vi "Constructor.vi"(7 "FP_Control_Flag":string="UI_", 8 "error in":errorcluster, 10 "UI_Ref":refnum<vi>, 11 "UI_Manager in":refnum<class "UI_Library.lvclass">) -> (0 "error out":errorcluster, 2 "UI_Queue":refnum<queue>, 3 "UI_Manager out":refnum<class "UI_Library.lvclass">)   [LabVIEW 2018, in "UI_Library.lvlib" / "UI_Library.lvclass"]
doc: "Initialize Class queue and properties"
uses:
  UI_Library.lvclass
  UI_Library.lvclass/UI_Library.ctl
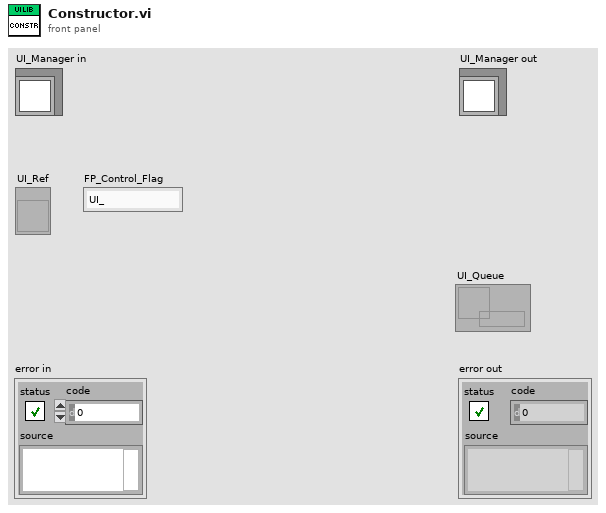
[diagram p1: front panel]
types:
  T1 = cluster{"UIEvent":string, "EventData":variant, "Register":bool}
  T2 = typedef "UI_Library.lvlib/UI_RefCluster.ctl" = cluster{"UI Ctrl Names":string[], "UI Ctrl DataType":T3[], "UI Ctrl Refs":refnum<vi>[]}
  T3 = typedef "NI_Data Type.lvlib/Data Type.ctl" = enum8{"Invalid Type", "Void", "I8", "I16", "I32", "I64", "U8", "U16", "U32", "U64", "Single Float", "Double Float", "Extended Float", "Single Complex", "Double Complex", "Extended Complex", "Enum U8", "Enum U16", "Enum U32", "Enum U64", "Single Float With Unit", "Double Float With Unit", "Extended Float With Unit", "Single Complex with Unit", "Double Complex with Unit", "Extended Complex with Unit", "Boolean", "String", "Path", "Picture", "Tag", "Array", "Cluster", "Variant", "LV Variant", "Waveform", "Timestamp", "Digital Waveform", "Digital Data", "ExpressData", "Refnum", "External Data", "VI", "Poly VI", "LabVIEW Class Instance", "Fixed Point", "Set Collection", "Map Collection"}
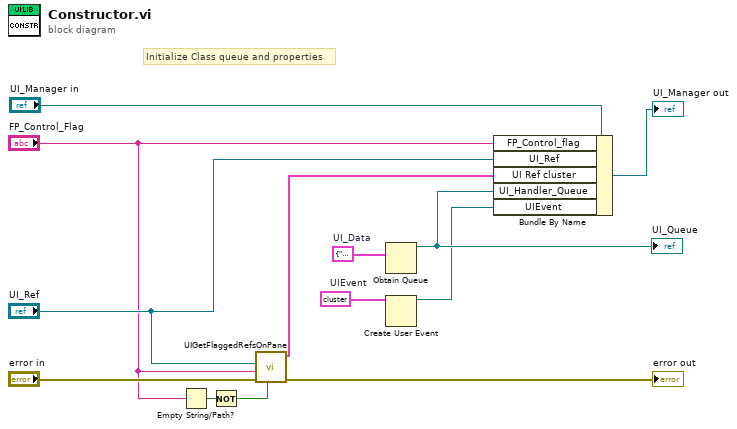
[diagram p0: block diagram]
diagram:
  w4 = T1 {"UIEvent"="", "EventData"=variant, "Register"=FALSE}  # UIEvent
  w12 = cluster{"cmd":string, "data":variant} {"cmd"="", "data"=variant}  # UI_Data
  # "Initialize Class queue and properties"
  n1 = Empty String/Path?(string/path="FP_Control_Flag") -> (empty?=w8:bool)
  n2 = Not(x=w8) -> (.not. x?=w6:bool)
  n3 = call "UIGetFlaggedRefsOnPane.vi"("Check Flag (T)"=w6, "error in"="error in", "Flag"="FP_Control_Flag", "VI Ref"="UI_Ref") -> ("error out"=→"error out":errorcluster, "UI Ref cluster out"=w5:T2)  [unwired: 6 in]
  n4 = Obtain Queue(element data type=w12) -> (queue out=w3:refnum<queue>)  [unwired: 4 in, 2 out]
  "UI_Queue" <- w3
  n5 = Create User Event(user event datatype=w4) -> (user event=w2:refnum<user-event>)  [unwired: 1 in, 1 out]
  n6 = Bundle By Name(cluster="UI_Manager in", "FP_Control_flag"="FP_Control_Flag", "UI_Ref"="UI_Ref", "UI Ref cluster"=w5, "UI_Handler_Queue"=w3, "UIEvent"=w2) -> (→"UI_Manager out":refnum<class "UI_Library.lvclass">)
